vi "CSGArrayToStr(cast).vi"(1 "CSG数组":csg[](array[numeric])) -> (0 "字符串":string)   [LabVIEW 2012]
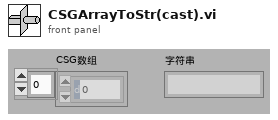
[diagram p1: front panel]
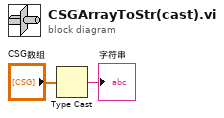
[diagram p0: block diagram]
diagram:
  n1 = Type Cast(x="CSG数组") -> (*(type *) &x=→"字符串":string)  [unwired: 1 in]
